vi "DAC_Xmit_order.vi"(2 "Order in":u64, 3 "FPGA VI Reference In":T1) -> (0 "error out":errorcluster, 1 "FPGA VI Reference Out":T1)   [LabVIEW 2013]
uses:
  fpga-bitfile-ref.ctl
  <vilib>/rvi/interface/common/niFpgaWaitOnOcc.vi
  <vilib>/Utility/error.llb/Error Cluster From Error Code.vi
  <vilib>/rvi/errors/niLvFpgaAdjustHostInterfaceError.vi
  <vilib>/RVI Host/nirviSupport.llb/nirviErrorClusterFromErrorCode.vi
  <vilib>/rvi/interface/nirviMethod/nirviMethod.xnode
  FPGA Bitfiles/FPGA_new_main_sbRIO_9612_10MHz_6us.lvbitx
  <vilib>/rvi/interface/nirviMethod/StockFPGA_InlinedMethodWaitForSingleIRQ.vi
  <vilib>/FPGAPlugInAG/sbRIO-9612/niLvFpga_WaitOnIrq_sbRIO-9612.vi
  <vilib>/FPGAPlugInAG/sbRIO-9612/niLvFpga_AcknowledgeIrq_sbRIO-9612.vi
  <vilib>/FPGAPlugInAG/sbRIO-9612/niLvFpga_WriteFifo_sbRIO-9612.vi
  <vilib>/rvi/errors/niLvFpgaMergeErrorWithErrorCode.vi
panel:
  in  "stop":bool
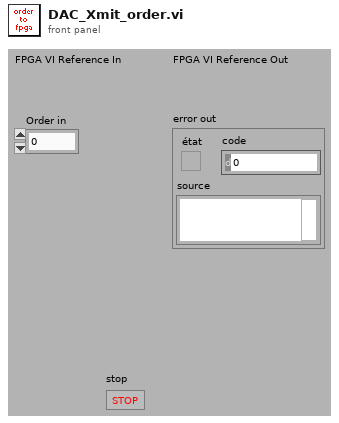
[diagram p1: front panel]
types:
  T1 = typedef "fpga-bitfile-ref.ctl" = refnum<k20>
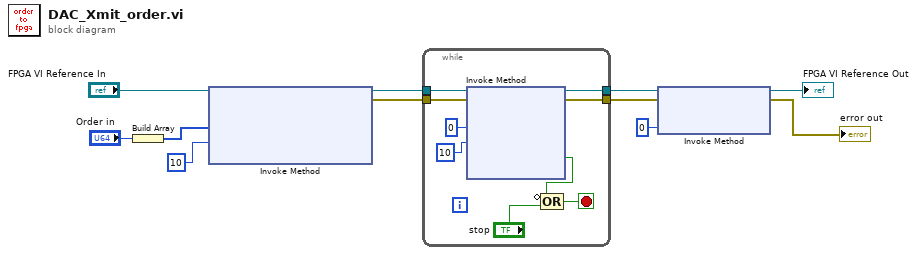
[diagram p0: block diagram]
diagram:
  n1 = Build Array("Order in") -> (w7:u64[])
  n2 = xnode "Invoke Method"("FPGA VI Reference In"="FPGA VI Reference In", "Data"=w7, "Timeout (ms)"=10) -> ("FPGA VI Reference Out"=w11:T1, "error out"=w10:errorcluster)  [unwired: 1 in, 1 out]
  n3 = while {
    tunnel: w11 -> [w20]
    tunnel: [w19] -> w4
    tunnel: [w18] -> w2
    tunnel: w10 -> [w17]
    stop <- w13 stop-if-true
    n4 = xnode "Invoke Method"("FPGA VI Reference In"=w20, "error in"=w17, "IRQ Number(s)"=0, "Timeout (ms)"=10) -> ("FPGA VI Reference Out"=w19:T1, "error out"=w18:errorcluster, "Timed Out"=w12:bool)  [unwired: 1 out]
    n5 = Compound Arithmetic op=OR(invert w12, "stop") -> (w13:bool)
  }
  n6 = xnode "Invoke Method"("FPGA VI Reference In"=w4, "error in"=w2, "IRQ Number(s)"=0) -> ("FPGA VI Reference Out"=→"FPGA VI Reference Out":T1, "error out"=→"error out":errorcluster)
